vi "vipm_InstallPackages.vi"(8 "error in (no error)":errorcluster, 11 "CommandLine":string[](array[string])=["ZAlign"]) -> (0 "error out":errorcluster, 2 "test details":string, 3 "output to action":string)   [LabVIEW 2014]
uses:
  <vilib>/JKI/VIPM API/command-line/support/Library Contents Cluster_vipm_api.ctl
  <userlib>/_OpenG.lib/array/array.llb/Index 1D Array Elements (String)__ogtk.vi
  <userlib>/_OpenG.lib/file/file.llb/File Exists - Scalar__ogtk.vi
  <userlib>/_OpenG.lib/array/array.llb/Filter 1D Array (String)__ogtk.vi
  <vilib>/JKI/VIPM API/VIPM API_vipm_api.lvlib
  _lvcicd/_lvcicd_support_2014.lvlib
panel:
  # "lava_lib_json_api-1.5.5.41"
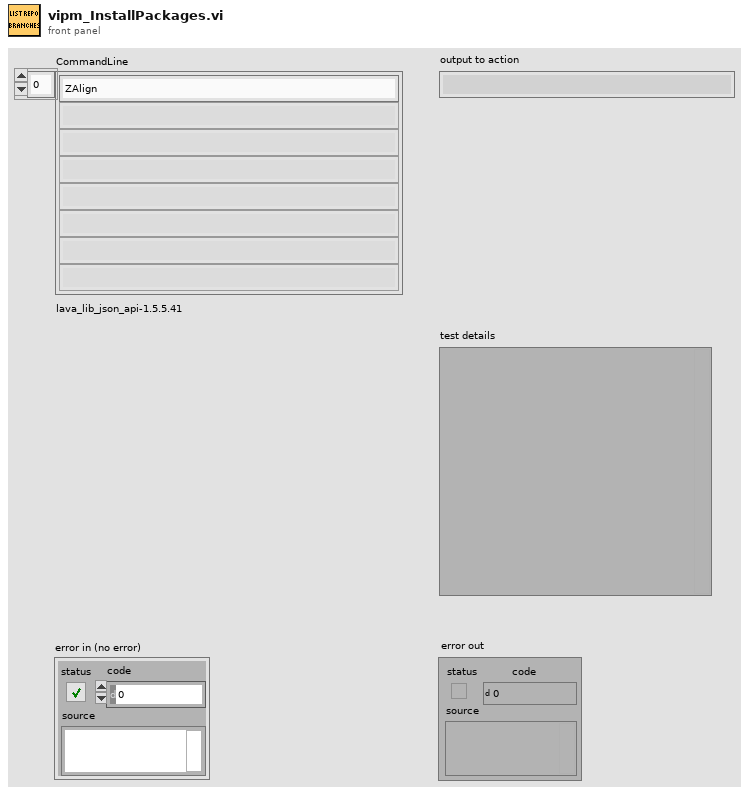
[diagram p1: front panel]
types:
  T1 = typedef "VIPM API_vipm_api.lvlib/Library Contents Cluster_vipm_api.ctl" = cluster{"Package Name":string, "Version":string, "Display Name":string, "Repository Name":string, "Company Name":string, "License Type":string, "Installed":bool, "Deprecated":bool, "Dependency or Conflict Problem":bool, "Downloaded":bool}
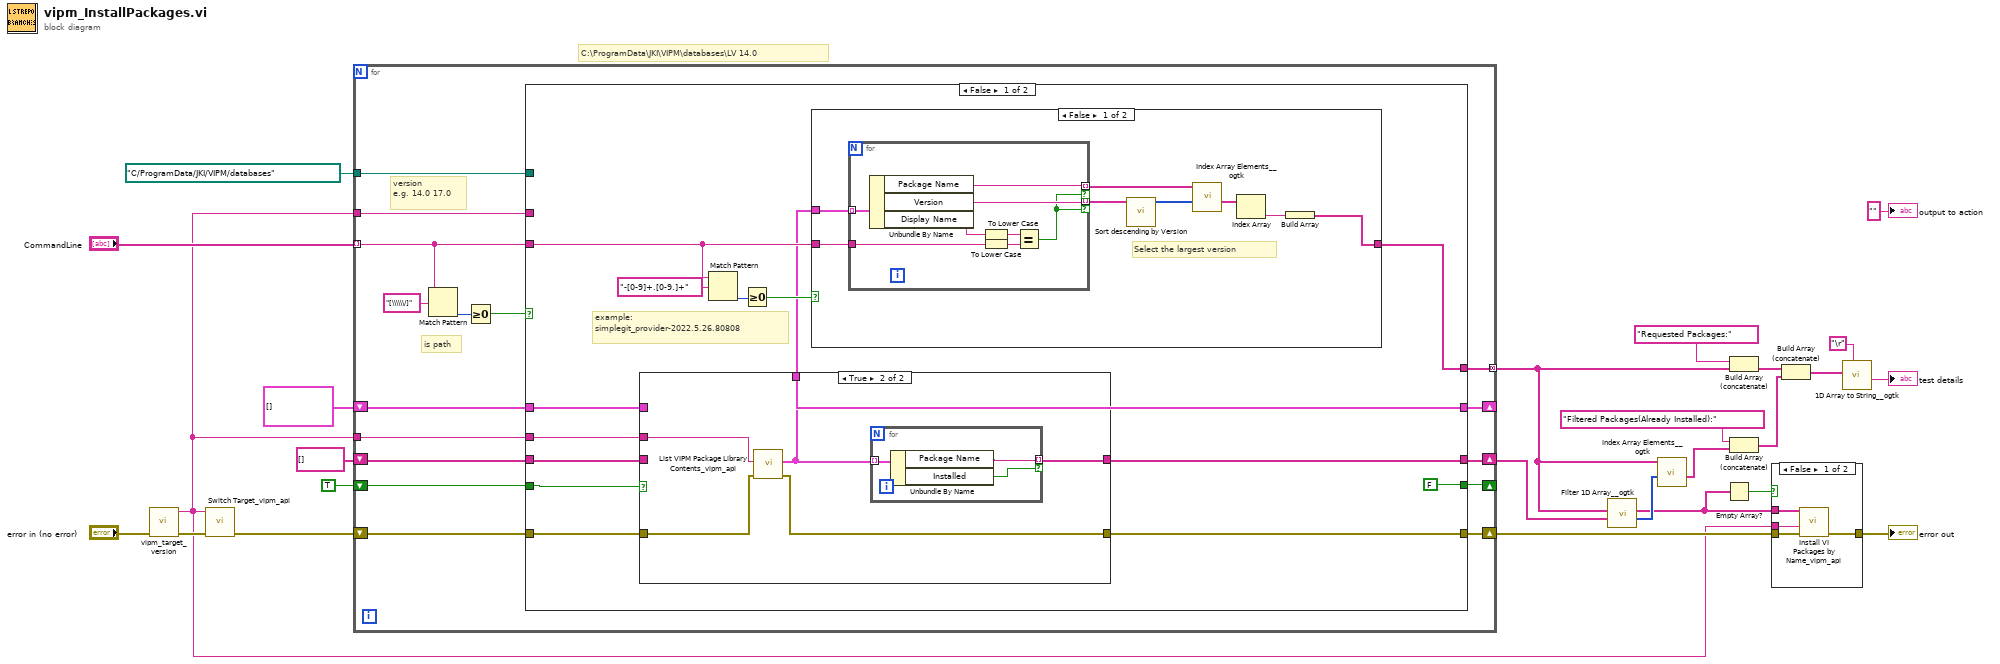
[diagram p0: block diagram]
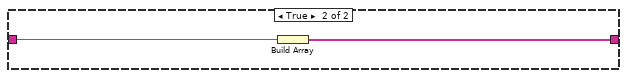
[diagram p4: hidden frame]
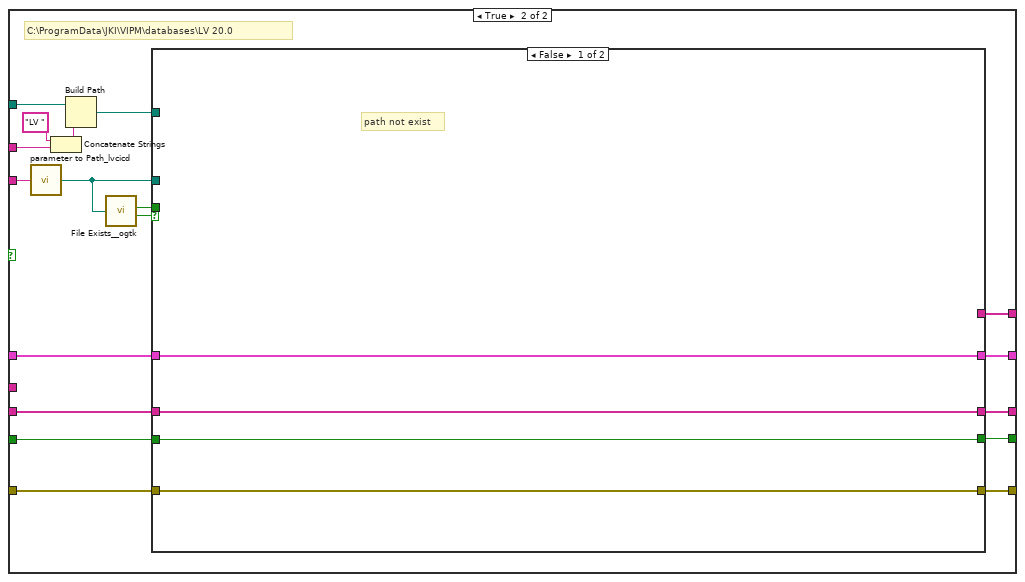
[diagram p5: hidden frame]
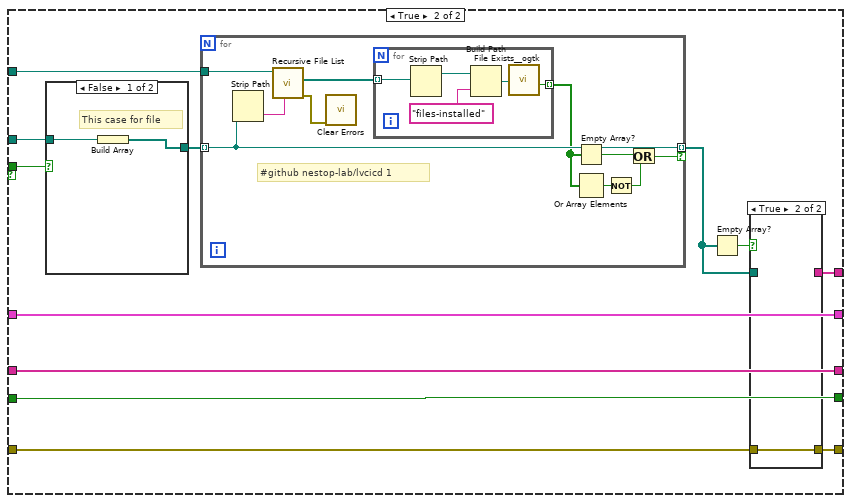
[diagram p6: hidden frame]
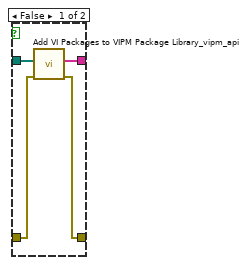
[diagram p7: hidden frame]
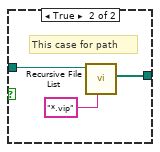
[diagram p8: hidden frame]
diagram:
  # "C:\\ProgramData\\JKI\\VIPM\\databases\\LV 14.0"
  n1 = call "vipm_target_version.vi"() -> ("vipm Taget version"=w2:string)  [unwired: 11 in]
  n2 = call <vilib>:"Switch Target_vipm_api.vi"("error in (no error)"="error in (no error)", "LabVIEW Version"=w2) -> ("error out"=w6:errorcluster)  [unwired: 9 in]
  n3 = for {
    tunnel: "CommandLine" -> [w34] mode=indexing
    tunnel: [w39] -> w17 mode=concatenating
    shift-right: [w38] -> w18
    shift-left: w6 -> [w40]
    tunnel: w2 -> [w33]
    tunnel: path "C:/ProgramData/JKI/VIPM/databases" -> [w32]
    shift-right: [w31] -> w4
    shift-left: string[] [] -> [w28]
    shift-right: [w29] -> _
    shift-left: TRUE -> [w30]
    tunnel: w2 -> [w27]
    shift-right: [w26] -> _
    shift-left: T1[] [] ("Library Contents []") -> [w25]
    # "version\ne.g. 14.0 17.0"
    # "is path"
    n4 = Match Pattern(string=w34, regular expression="[\\\\\\/]") -> (offset past match=w36:i32)  [unwired: 1 in, 3 out]
    n5 = Greater Or Equal To 0?(x=w36) -> (x >= 0?=w35:bool)
    n6 = case shown="False" w35 {
      tunnel: w40 -> [w46 w101]
      tunnel: [w54 w100] -> w39
      tunnel: [w45 w99] -> w38
      tunnel: w34 -> [w52 w98]
      tunnel: w33 -> [_ w94]
      tunnel: w32 -> [_ w91]
      tunnel: [w49 w87] -> w31
      tunnel: w30 -> [w44 w88]
      tunnel: [FALSE w89] -> w29
      tunnel: w28 -> [w41 w86]
      tunnel: w27 -> [w47 _]
      tunnel: [w43 w85] -> w26
      tunnel: w25 -> [w42 w84]
      frame False {
        # "example:\nsimplegit_provider-2022.5.26.80808"
        n7 = case shown="True" w44 {
          tunnel: [w56 w62] -> w49
          tunnel: w47 -> [_ w61]
          tunnel: w46 -> [w55 w60]
          tunnel: [w55 w59] -> w45
          tunnel: [w57 w58] -> w43
          tunnel: w42 -> [w57 _]
          tunnel: w41 -> [w56 _]
          frame False {
          }
          frame True {
            n8 = call <vilib>:"List VIPM Package Library Contents_vipm_api.vi"("error in (no error)"=w60, "LabVIEW Version"=w61) -> ("error out"=w59:errorcluster, "Library Contents []"=w58:T1[])  [unwired: 7 in, 1 out]
            n9 = for {
              tunnel: w58 -> [w65] mode=indexing
              tunnel: [w64] -> w62 mode=indexing if=w63
              n10 = Unbundle By Name(w65) -> ("Package Name"=w64:string, "Installed"=w63:bool)
            }
          }
        }
        n11 = Match Pattern(string=w52, regular expression="-[0-9]+.[0-9.]+") -> (offset past match=w51:i32)  [unwired: 1 in, 3 out]
        n12 = Greater Or Equal To 0?(x=w51) -> (x >= 0?=w50:bool)
        n13 = case shown="False" w50 {
          tunnel: w43 -> [w73 _]
          tunnel: [w67 w82] -> w54
          tunnel: w52 -> [w66 w83]
          frame False {
            # "Select the largest version"
            n14 = for {
              tunnel: w73 -> [w81] mode=indexing
              tunnel: w66 -> [w79]
              tunnel: [w78] -> w72 mode=indexing if=w76
              tunnel: [w77] -> w71 mode=indexing if=w76
              n15 = Unbundle By Name(w81) -> ("Package Name"=w77:string, "Version"=w78:string, "Display Name"=w80:string)
              n16 = To Lower Case(string=w80) -> (all lower case string=w75:string)
              n17 = To Lower Case(string=w79) -> (all lower case string=w74:string)
              n18 = Equal?(x=w75, y=w74) -> (x = y?=w76:bool)
            }
            n19 = call "Sort descending by Version.vi"("Array"=w72) -> ("Sorted Pointers"=w70:i32[])  [unwired: 10 in]
            n20 = call-poly <userlib>:"Index Array Elements__ogtk.vi"("indices"=w70, "array"=w71) -> ("elements"=w69:string[])  [unwired: 9 in]
            n21 = Index Array(array=w69) -> (element=w68:string)  [unwired: 1 in]
            n22 = Build Array(w68) -> (w67:string[])
          }
          frame True {
            n23 = Build Array(w83) -> (w82:string[])
          }
        }
      }
      frame True {
        # "C:\\ProgramData\\JKI\\VIPM\\databases\\LV 20.0"
        n24 = call "parameter to Path_lvcicd.vi"("String"=w98) -> ("Path"=w97:path)
        n25 = Concatenate Strings("LV " ("string"), w94) -> (w92:string)
        n26 = Build Path(base path=w91, name or relative path=w92) -> (appended path=w90:path)
        n27 = call-poly <userlib>:"File Exists__ogtk.vi"("file path"=w97) -> ("is directory"=w95:bool, "exists"=w96:bool)  [unwired: 6 in]
        n28 = case shown="False" w96 {
          tunnel: w101 -> [w105 w117]
          tunnel: [_ w116] -> w100
          tunnel: [w105 w115] -> w99
          tunnel: w97 -> [_ w114]
          tunnel: w95 -> [_ w113]
          tunnel: w90 -> [_ w111]
          tunnel: [w104 w108] -> w89
          tunnel: w88 -> [w104 w108]
          tunnel: [w103 w107] -> w87
          tunnel: w86 -> [w103 w107]
          tunnel: [w102 w106] -> w85
          tunnel: w84 -> [w102 w106]
          frame False {
            # "path not exist"
          }
          frame True {
            n29 = case shown="False" w113 {
              tunnel: [w139 w140] -> w112
              tunnel: w114 -> [w138 w142]
              frame False {
                # "This case for file"
                n30 = Build Array(w138) -> (w139:path[])
              }
              frame True {
                # "This case for path"
                n31 = call <vilib>:"Recursive File List.vi"("pattern"="*.vip", "Folder Path"=w142) -> ("All Files in Dir"=w140:path[])  [unwired: 5 in, 4 out]
              }
            }
            n32 = for {
              tunnel: [w132] -> w110 mode=indexing if=w126
              tunnel: w112 -> [w132] mode=indexing
              tunnel: w111 -> [w131]
              # "#github nestop-lab/lvcicd 1"
              n33 = Strip Path(path=w132) -> (name=w130:string)  [unwired: 1 out]
              n34 = call <vilib>:"Recursive File List.vi"("pattern"=w130, "Folder Path"=w131) -> ("error out"=w123:errorcluster, "All Files in Dir"=w129:path[])  [unwired: 5 in, 3 out]
              n35 = call <vilib>:"Clear Errors.vi"("error in (no error)"=w123) -> ()  [unwired: 5 in, 2 out]
              n36 = for {
                tunnel: w129 -> [w137] mode=indexing
                tunnel: [w133] -> w128 mode=indexing
                n37 = Strip Path(path=w137) -> (stripped path=w136:path)  [unwired: 1 out]
                n38 = Build Path(base path=w136, name or relative path="files-installed") -> (appended path=w134:path)
                n39 = call-poly <userlib>:"File Exists__ogtk.vi"("file path"=w134) -> ("exists"=w133:bool)  [unwired: 6 in, 1 out]
              }
              n40 = Empty Array?(array=w128) -> (empty?=w125:bool)
              n41 = Or Array Elements(Boolean array=w128) -> (logical OR=w127:bool)
              n42 = Not(x=w127) -> (.not. x?=w124:bool)
              n43 = Or(x=w125, y=w124) -> (x .or. y?=w126:bool)
            }
            n44 = Empty Array?(array=w110) -> (empty?=w109:bool)
            n45 = case shown="True" w109 {
              tunnel: w117 -> [w121 w122]
              tunnel: [w120 _] -> w116
              tunnel: [w119 w122] -> w115
              tunnel: w110 -> [w118 _]
              frame False {
                n46 = call <vilib>:"Add VI Packages to VIPM Package Library_vipm_api.vi"("error in (no error)"=w121, "Packages to add to VIPM Library (vipc,vip,ogp)"=w118) -> ("error out"=w119:errorcluster, "Package Names Added"=w120:string[])  [unwired: 8 in]
              }
              frame True {
              }
            }
          }
        }
      }
    }
  }
  n47 = call-poly <userlib>:"Filter 1D Array__ogtk.vi"("items to filter"=w4, "array"=w17) -> ("filtered item indices"=w16:i32[], "filtered array"=w9:string[])  [unwired: 4 in]
  n48 = call-poly <userlib>:"Index Array Elements__ogtk.vi"("indices"=w16, "array"=w17) -> ("elements"=w13:string[])  [unwired: 9 in]
  n49 = Empty Array?(array=w9) -> (empty?=w8:bool)
  n50 = Build Array (concatenate)("Requested Packages:" ("output to action"), w17) -> (w15:string[])
  n51 = Build Array (concatenate)("Filtered Packages(Already Installed):" ("output to action"), w13) -> (w10:string[])
  n52 = case shown="False" w8 {
    tunnel: [w146 w147] -> w24
    tunnel: w18 -> [w145 w147]
    tunnel: w2 -> [w144 _]
    tunnel: w9 -> [w143 _]
    frame False {
      n53 = call <vilib>:"Install VI Packages by Name_vipm_api.vi"("error in (no error)"=w145, "LabVIEW Version"=w144, "Package Names to Install []"=w143) -> ("error out"=w146:errorcluster)  [unwired: 8 in]
    }
    frame True {
    }
  }
  "error out" <- w24
  n54 = Build Array (concatenate)(w15, w10) -> (w11:string[])
  n55 = call <userlib>:"1D Array to String__ogtk.vi"("delimiter (Tab)"="\r" ("Carriage Return Constant"), "Array of Strings"=w11) -> ("delimited string"=→"test details":string)  [unwired: 9 in]
  "output to action" <- "" ("output to action")
